vi "Image from position spec.vi"(7 "Timelapse image":T1, 9 "Image position":T2=enum."Top right", 10 "Stitch layout spec":T4, 11 "Cam videos cluster":T3 {"Vid4 Rel time (ms)" format="%.0f ms"; "Vid3 Rel time (ms)" format="%.0f ms"; "Vid2 Rel time (ms)" format="%.0f ms"; "Vid1 Rel time (ms)" format="%.0f ms"}) -> (3 "Selected image":T1)   [LabVIEW 2013]
uses:
  Cam video sync/Typedefs/Stitch layout spec cluster.ctl
  Typedefs/Image stitching positions.ctl
  <vilib>/vision/Image Controls.llb/IMAQ Image.ctl
  Cam video sync/Typedefs/Cam videos cluster.ctl
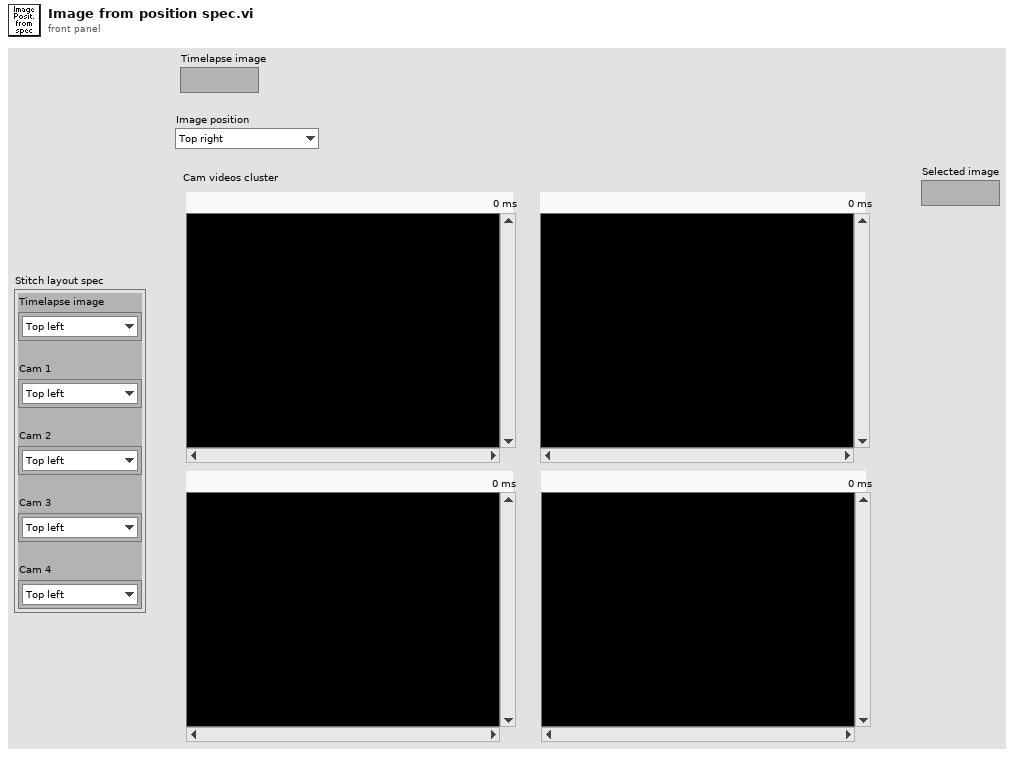
[diagram p1: front panel]
types:
  T1 = typedef "IMAQ Image.ctl" = refnum<image>
  T2 = typedef "Image stitching positions.ctl" = enum16{"Top left", "Top right", "Bottom left", "Bottom right", "Not used"}
  T3 = typedef "Cam videos cluster.ctl" = cluster{"Vid 1":T1, "Vid 2":T1, "Vid 3":T1, "Vid 4":T1, "Vid1 Rel time (ms)":u32, "Vid2 Rel time (ms)":u32, "Vid3 Rel time (ms)":u32, "Vid4 Rel time (ms)":u32}
  T4 = typedef "Stitch layout spec cluster.ctl" = cluster{"Timelapse image":cluster{"Image position":T2}, "Cam 1":cluster{"Image position":T2}, "Cam 2":cluster{"Image position":T2}, "Cam 3":cluster{"Image position":T2}, "Cam 4":cluster{"Image position":T2}}
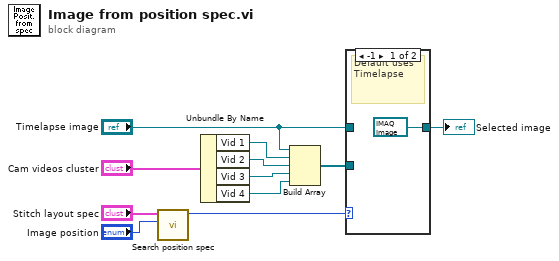
[diagram p0: block diagram]
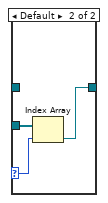
[diagram p2: hidden frame]
diagram:
  n1 = call "Search position spec.vi"("Image position"="Image position", "Stitch layout spec"="Stitch layout spec") -> ("index of element"=w5:i32)  [unwired: 9 in]
  n2 = Unbundle By Name("Cam videos cluster") -> ("Vid 1"=w4:T1, "Vid 2"=w9:T1, "Vid 3"=w8:T1, "Vid 4"=w2:T1)
  n3 = Build Array("Timelapse image", w4, w9, w8, w2) -> (w7:T1[])
  n4 = case shown="-1" w5 {
    selector: w5 -> [_ w13]
    tunnel: w7 -> [_ w15]
    tunnel: [T1 refnum ("Vid 4") w14] -> w6
    tunnel: "Timelapse image" -> [_ _]
    frame -1 {
      # "Default uses Timelapse"
    }
    frame Default {
      n5 = Index Array(array=w15, index=w13) -> (element=w14:T1)
    }
  }
  "Selected image" <- w6
